vi "get tracking data info.vi"(8 "error in (no error)":errorcluster caption="에러 입력(에러 없음)", 11 "Auto Tracking Wave 입력":refnum<class "Auto Track Wave.lvclass">) -> (0 "error out":errorcluster caption="에러 출력", 1 "warning":bool, 2 "wave length":dbl, 3 "Auto Tracking Wave 출력":refnum<class "Auto Track Wave.lvclass">, 4 "brake wave freq":dbl)   [LabVIEW 2020, in "Auto Track Wave.lvclass"]
uses:
  Auto Track Wave.lvclass
  Waveform Obj/Waveform Obj.lvclass/Waveform Obj.ctl
  Waveform Gen/Waveform Gen.lvclass/Waveform Gen.ctl
  Auto Track Wave.lvclass/Auto Track Wave.ctl
  Waveform Obj/Accessors/Read sampling rate.vi
  Waveform Gen/Accessors/Read frequency.vi
  Accessors/Read zxd time.vi
  Accessors/Read null time.vi
  Accessors/Read gnd time.vi
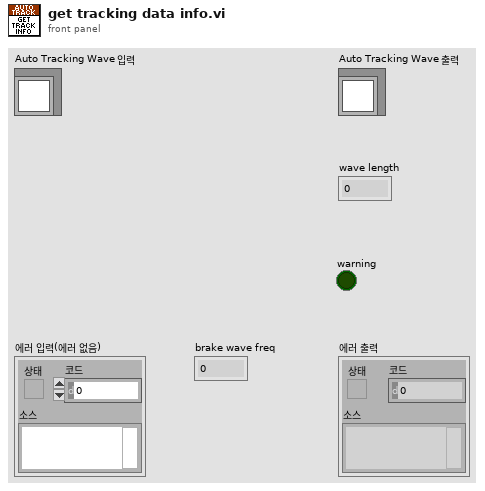
[diagram p1: front panel]
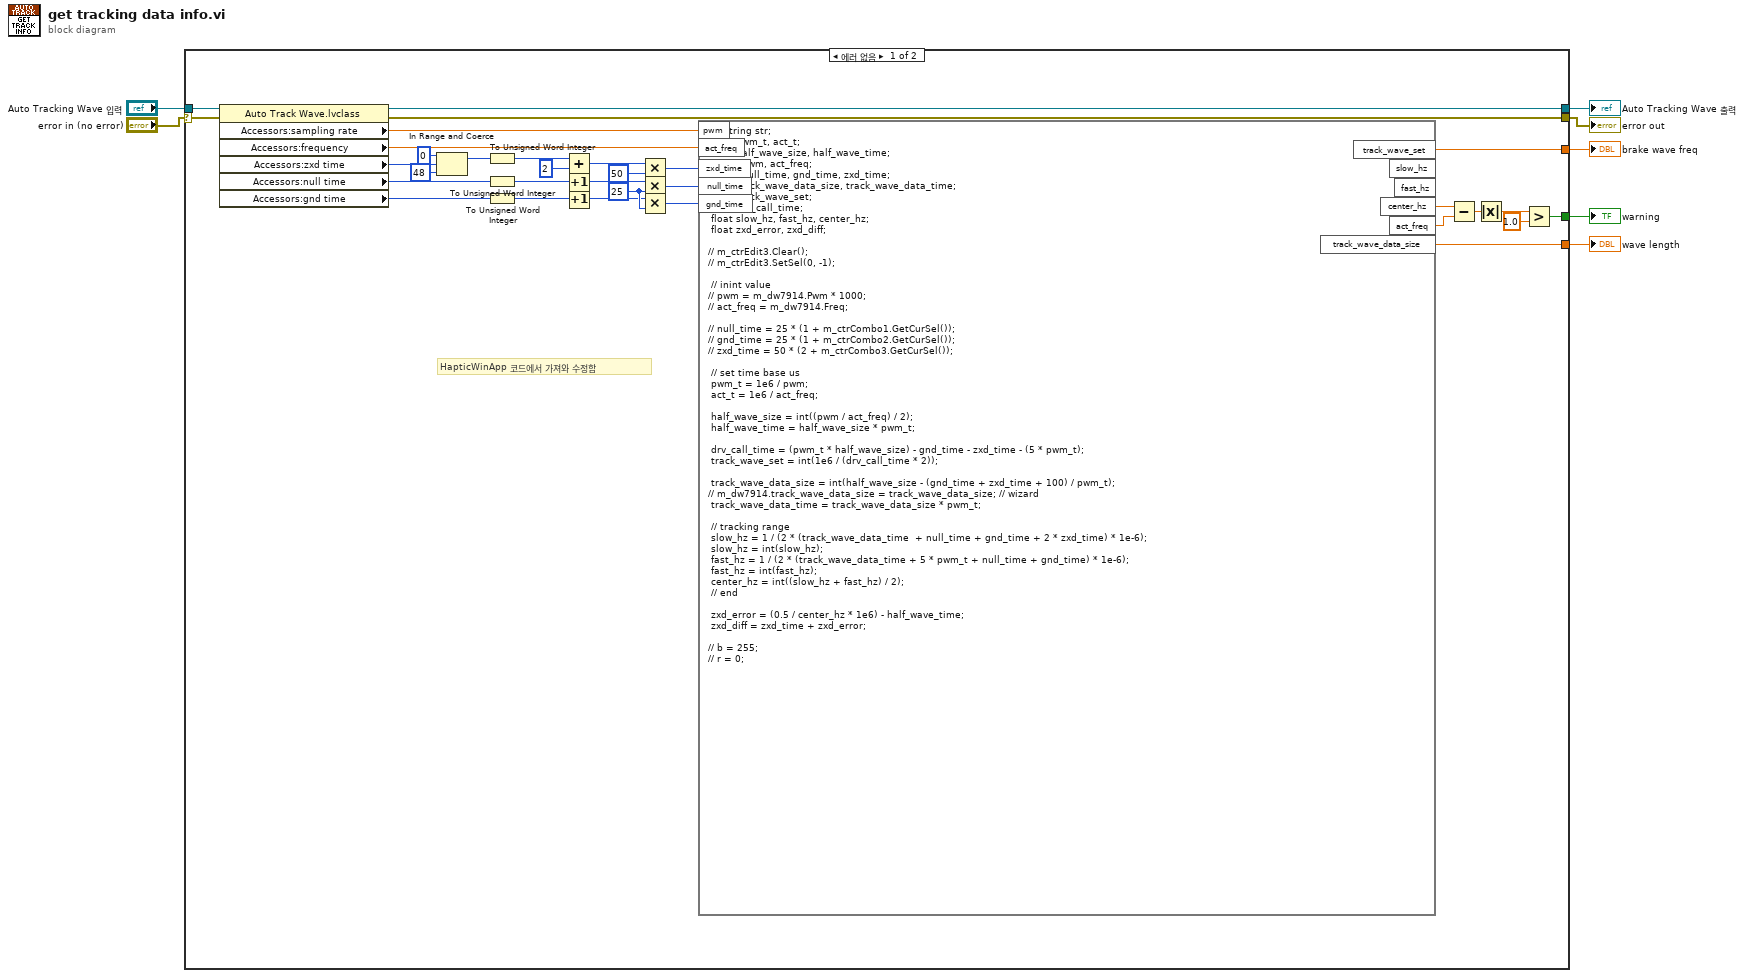
[diagram p0: block diagram]
diagram:
  n1 = case shown="에러 없음" "error in (no error)" {
    selector: "error in (no error)" -> [w39 w41]
    tunnel: [w36 w41] -> w4
    tunnel: [w37 w40] -> w6
    tunnel: "Auto Tracking Wave 입력" -> [w38 w40]
    tunnel: [w31 _] -> w3
    tunnel: [w9 _] -> w2
    tunnel: [w8 _] -> w1
    frame No Error {
      w28 = u16 25 ("y")
      # "HapticWinApp 코드에서 가져와 수정함"
      n2 = property class="Auto Track Wave.lvclass"(reference=w38, error in=w39) -> (reference out=w37:refnum<class "Auto Track Wave.lvclass">, error out=w36:errorcluster, "Accessors:sampling rate"=w35:dbl, "Accessors:frequency"=w34:dbl, "Accessors:zxd time"=w25:u8, "Accessors:null time"=w33:u8, "Accessors:gnd time"=w32:u8)
      n3 = In Range and Coerce(upper limit=u8 0 ("상위 리미트"), x=w25, lower limit=u8 48 ("하위 리미트")) -> (coerced(x)=w24:u8)  [unwired: 1 out]
      n4 = To Unsigned Word Integer(number=w24) -> (unsigned 16bit integer=w22:u16)
      n5 = To Unsigned Word Integer(number=w33) -> (unsigned 16bit integer=w21:u16)
      n6 = To Unsigned Word Integer(number=w32) -> (unsigned 16bit integer=w20:u16)
      n7 = Add(x=w22, y=u16 2) -> (x+y=w18:u16)
      n8 = Increment(x=w21) -> (x+1=w17:u16)
      n9 = Increment(x=w20) -> (x+1=w16:u16)
      n10 = Multiply(x=w18, y=u16 50) -> (x*y=w19:u16)
      n11 = Multiply(x=w17, y=w28) -> (x*y=w30:u16)
      n12 = Multiply(x=w16, y=w28) -> (x*y=w29:u16)
      n13 = formula code="//\tCString str;\n\tfloat pwm_t, act_t;\n\tfloat half_wave_size, half_wave_time;\n//\tfloat pwm, act_freq;\n//\tfloat null_time, gnd_time, zxd_time;\n\tfloat track_wave_data_size, track_wave_data_time;\n\tfloat track_wave_set;\n\tfloat drv_call_time;\n\tfloat slow_hz, fast_hz, center_hz;\n\tfloat zxd_error, zxd_diff;\n\n//\tm_ctrEdit3.Clear();\n//\tm_ctrEdit3.SetSel(0, -1);\n\n\t// inint value\n//\tpwm = m_dw7914.Pwm * 1000;\n//\tact_freq = m_dw7914.Freq;\n\n//\tnull_time = 25 * (1 + m_ctrCombo1.GetCurSel());\n//\tgnd_time = 25 * (1 + m_ctrCombo2.GetCurSel());\n//\tzxd_time = 50 * (2 + m_ctrCombo3.GetCurSel());\n\n\t// set time base us\n\tpwm_t = 1e6 / pwm;\n\tact_t = 1e6 / act_freq;\n\n\thalf_wave_size = int((pwm / act_freq) / 2);\n\thalf_wave_time = half_wave_size * pwm_t;\n\n\tdrv_call_time = (pwm_t * half_wave_size) - gnd_time - zxd_time - (5 * pwm_t);\n\ttrack_wave_set = int(1e6 / (drv_call_time * 2));\n\n\ttrack_wave_data_size = int(half_wave_size - (gnd_time + zxd_time + 100) / pwm_t);\n//\tm_dw7914.track_wave_data_size = track_wave_data_size;\t// wizard\n\ttrack_wave_data_time = track_wave_data_size * pwm_t;\n\n\t// tracking range\n\tslow_hz = 1 / (2 * (track_wave_data_time  + null_time + gnd_time + 2 * zxd_time) * 1e-6);\n\tslow_hz = int(slow_hz);\n\tfast_hz = 1 / (2 * (track_wave_data_time + 5 * pwm_t + null_time + gnd_time) * 1e-6);\n\tfast_hz = int(fast_hz);\n\tcenter_hz = int((slow_hz + fast_hz) / 2);\n\t// end\n\n\tzxd_error = (0.5 / center_hz * 1e6) - half_wave_time;\n\tzxd_diff = zxd_time + zxd_error;\n\n//\tb = 255;\n//\tr = 0;"("pwm"=w35, "act_freq"=w34, "null_time"=w30, "gnd_time"=w29, "zxd_time"=w19) -> ("track_wave_set"=w8:dbl, "center_hz"=w13:dbl, "act_freq"=w14:dbl, "track_wave_data_size"=w31:dbl)  [unwired: 2 out]
      n14 = Subtract(x=w13, y=w14) -> (x-y=w12:dbl)
      n15 = Absolute Value(x=w12) -> (abs(x)=w11:dbl)
      n16 = Greater?(x=w11, y=1.0) -> (0:w9:bool)
    }
    frame Error {
    }
  }
  "error out" <- w4
  "Auto Tracking Wave 출력" <- w6
  "wave length" <- w3
  "warning" <- w2
  "brake wave freq" <- w1
